vi "WriteErrorMessage.vi"(8 "error in (no error)":errorcluster, 9 "Node qualifier":string, 10 "GObj Refnum":refnum<vi>, 11 "Blacklist in":refnum<class "Blacklist.lvclass">) -> (0 "error out":errorcluster, 2 "dup GObj Refnum":refnum<vi>, 3 "Blacklist out":refnum<class "Blacklist.lvclass">)   [LabVIEW 2014, in "lvbuildsecurity.lvlib" / "Blacklist.lvclass"]
uses:
  Blacklist.lvclass
  Blacklist.lvclass/Blacklist.ctl
  lvbuildsecurity.lvlib
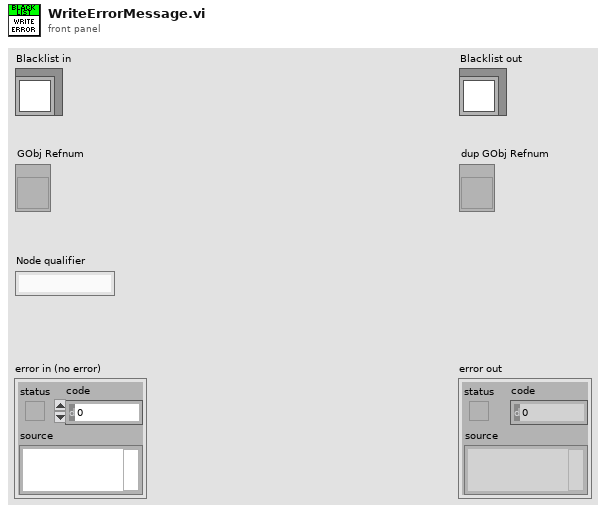
[diagram p1: front panel]
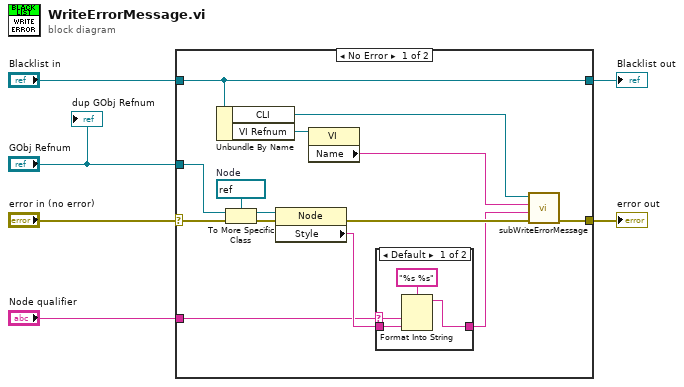
[diagram p0: block diagram]
diagram:
  n1 = case shown="No Error" "error in (no error)" {
    selector: "error in (no error)" -> [w20 w27]
    tunnel: [w10 w27] -> w5
    tunnel: [w15 w26] -> w3
    tunnel: "Blacklist in" -> [w15 w26]
    tunnel: "GObj Refnum" -> [w19 _]
    tunnel: "Node qualifier" -> [w12 _]
    frame No Error {
      w18 = refnum<vi> refnum  # Node
      n2 = Unbundle By Name(w15) -> ("CLI"=w9:refnum<class "CLI.lvclass">, "VI Refnum"=w14:refnum<vi>)
      n3 = To More Specific Class(target class=w18, reference=w19, error in=w20) -> (specific class reference=w16:refnum<vi>, error out=w17:errorcluster)
      n4 = property class="Node"(reference=w16, error in=w17) -> (error out=w11:errorcluster, "Style"=w13:string)  [unwired: 1 out]
      n5 = property class="VI"(reference=w14) -> ("Name"=w8:string)  [unwired: 1 in, 2 out]
      n6 = case shown="Default" w12 {
        selector: w12 -> [w21 _]
        tunnel: w13 -> [w22 w25]
        tunnel: [w24 w25] -> w7
        frame Default {
          n7 = Format Into String(format string="%s %s", w21, w22) -> (resulting string=w24:string)  [unwired: 2 in, 1 out]
        }
        frame "" {
        }
      }
      n8 = call "subWriteErrorMessage.vi"("error in (no error)"=w11, "Restricted Object"=w7, "VI Name"=w8, "CLI in"=w9) -> ("error out"=w10:errorcluster)  [unwired: 6 in, 1 out]
    }
    frame Error {
    }
  }
  "error out" <- w5
  "Blacklist out" <- w3
  "dup GObj Refnum" <- "GObj Refnum"
